vi "Video read with led for 3 part drum.vi"() -> ()   [LabVIEW 2009]
uses:
  <vilib>/vision/Image Controls.llb/IMAQ Image.ctl
  <vilib>/Instr/_visa.llb/VISA Configure Serial Port (Instr).vi
  <vilib>/Analysis/3filter.llb/Filter Passband Type.ctl
  <vilib>/Analysis/3filter.llb/Butterworth Filter (DBL).vi
  <vilib>/vision/NI_Vision_Development_Module.lvlib
  <vilib>/Analysis/NI_AALBase.lvlib
panel:
  in  "ROI Descriptor (Line Profile 2) 3":T1={"Global Rectangle"=[406, 309, 423, 383], "Contours"=[{"ID"=enum."External", "Type"=2, "Coordinates"=[422, 382, 406, 309]}]} {"Contours"."Type" items=["No Selection", "Point", "Line", "Rectangle", "Oval", "Polygon", "Freehand Region", "Annulus", "Unused2", "Unused3", "Broken Line", "Freehand Line", "Rotated Rectangle"]}
  in  "low  3":dbl=0.12500000000000006 format="%0.4f"
  out "Waveform Green":dbl[](graph)
  out "LED Green":bool
  in  "sampling 3":dbl=1.0 format="%0.2f"
  in  "high 3":dbl=60.0 format="%0.2f"
  in  "ROI Descriptor (Line Profile 2)":T1={"Global Rectangle"=[342, 292, 349, 377], "Contours"=[{"ID"=enum."External", "Type"=2, "Coordinates"=[342, 376, 348, 292]}]} {"Contours"."Type" items=["No Selection", "Point", "Line", "Rectangle", "Oval", "Polygon", "Freehand Region", "Annulus", "Unused2", "Unused3", "Broken Line", "Freehand Line", "Rotated Rectangle"]}
  out "Blue Line":T1={"Global Rectangle"=[168, 264, 180, 378], "Contours"=[{"ID"=enum."External", "Type"=2, "Coordinates"=[168, 377, 179, 264]}]} {"Contours"."Type" items=["No Selection", "Point", "Line", "Rectangle", "Oval", "Polygon", "Freehand Region", "Annulus", "Unused2", "Unused3", "Broken Line", "Freehand Line", "Rotated Rectangle"]}
  in  "ROI Descriptor (Line Profile 1) 2":T1={"Global Rectangle"=[376, 303, 382, 378], "Contours"=[{"ID"=enum."External", "Type"=2, "Coordinates"=[376, 303, 381, 377]}]} {"Contours"."Type" items=["No Selection", "Point", "Line", "Rectangle", "Oval", "Polygon", "Freehand Region", "Annulus", "Unused2", "Unused3", "Broken Line", "Freehand Line", "Rotated Rectangle"]}
  out "cluster":T2
  in  "baud rate (9600)":u32=9600
  in  "VISA resource name":refnum<visa-resource-name>
  out "number":u32
  out "decimal integer string":string
  out "Image Dst Out":T3
  out "Yellow Line":T1={"Global Rectangle"=[243, 262, 261, 384], "Contours"=[{"ID"=enum."External", "Type"=2, "Coordinates"=[260, 383, 243, 262]}]} {"Contours"."Type" items=["No Selection", "Point", "Line", "Rectangle", "Oval", "Polygon", "Freehand Region", "Annulus", "Unused2", "Unused3", "Broken Line", "Freehand Line", "Rotated Rectangle"]}
  in  "low  2":dbl=0.12500000000000006 format="%0.4f"
  in  "high 2":dbl=60.0 format="%0.2f"
  in  "sampling 2":dbl=1.0 format="%0.2f"
  out "LED RED":bool
  out "Waveform Yellow":dbl[](graph)
  in  "playtime":dbl=30.0
  out "Frame Number":i32
  in  "Frame Start":i32=2400
  out "LED BLUE":bool
  in  "low":dbl=0.12500000000000006 format="%0.4f"
  out "Waveform Blue":dbl[](graph)
  in  "high":dbl=60.0 format="%0.2f"
  in  "sampling":dbl=1.0 format="%0.2f"
  out "Image":T3(plugin-control)
  in  "stop":bool
  in  "AVI Path":path
  # "RED"
  # "BLUE"
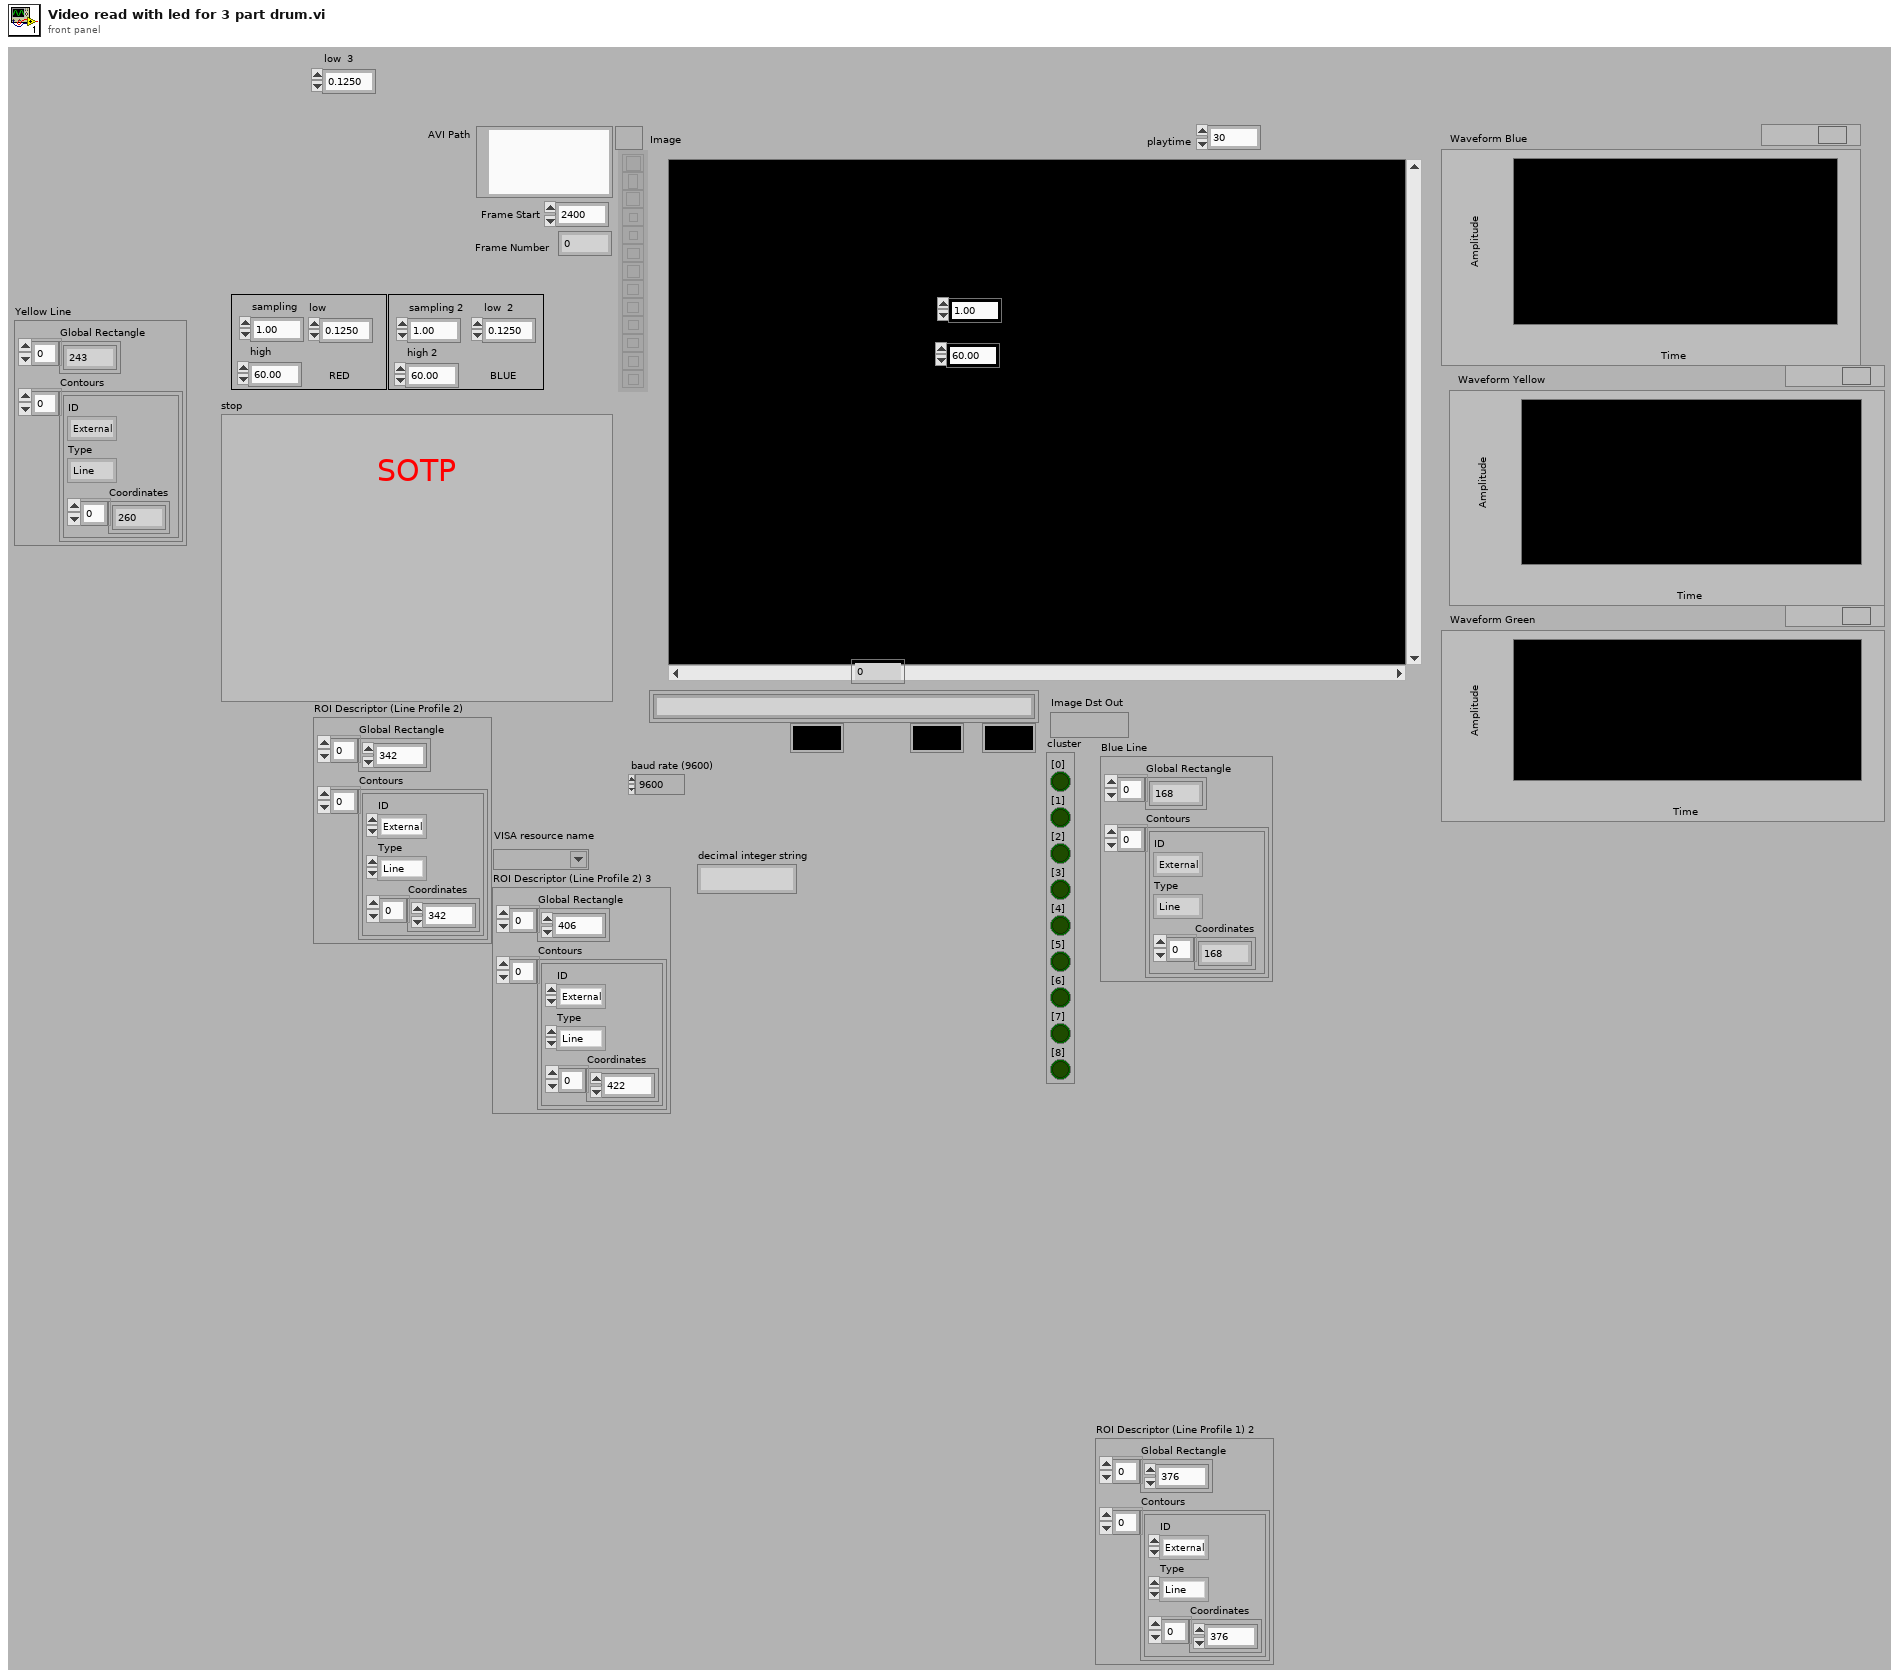
[diagram p1: front panel]
types:
  T1 = cluster{"Global Rectangle":i32[], "Contours":cluster{"ID":enum32{"External", "Internal"}, "Type":u32, "Coordinates":i32[]}[]}
  T2 = cluster{"[0]":bool, "[1]":bool, "[2]":bool, "[3]":bool, "[4]":bool, "[5]":bool, "[6]":bool, "[7]":bool, "[8]":bool}
  T3 = typedef "IMAQ Image.ctl" = refnum<image>
  T4 = typedef "NI_AALBase.lvlib/Filter Passband Type.ctl" = enum32{"Lowpass", "Highpass", "Bandpass", "Bandstop"}
  T5 = cluster{"Left":i32, "Top":i32, "Right":i32, "Bottom":i32}
  T6 = typedef "Image Type" = u32
  T7 = typedef "AviRefnum.ctl" = refnum<k1>
  T8 = cluster{"ID":enum32{"External", "Internal"}, "Type":u32, "Coordinates":i32[]}[]
  T9 = cluster{"ID":enum32{"External", "Internal"}, "Type":u32, "Coordinates":i32[]}
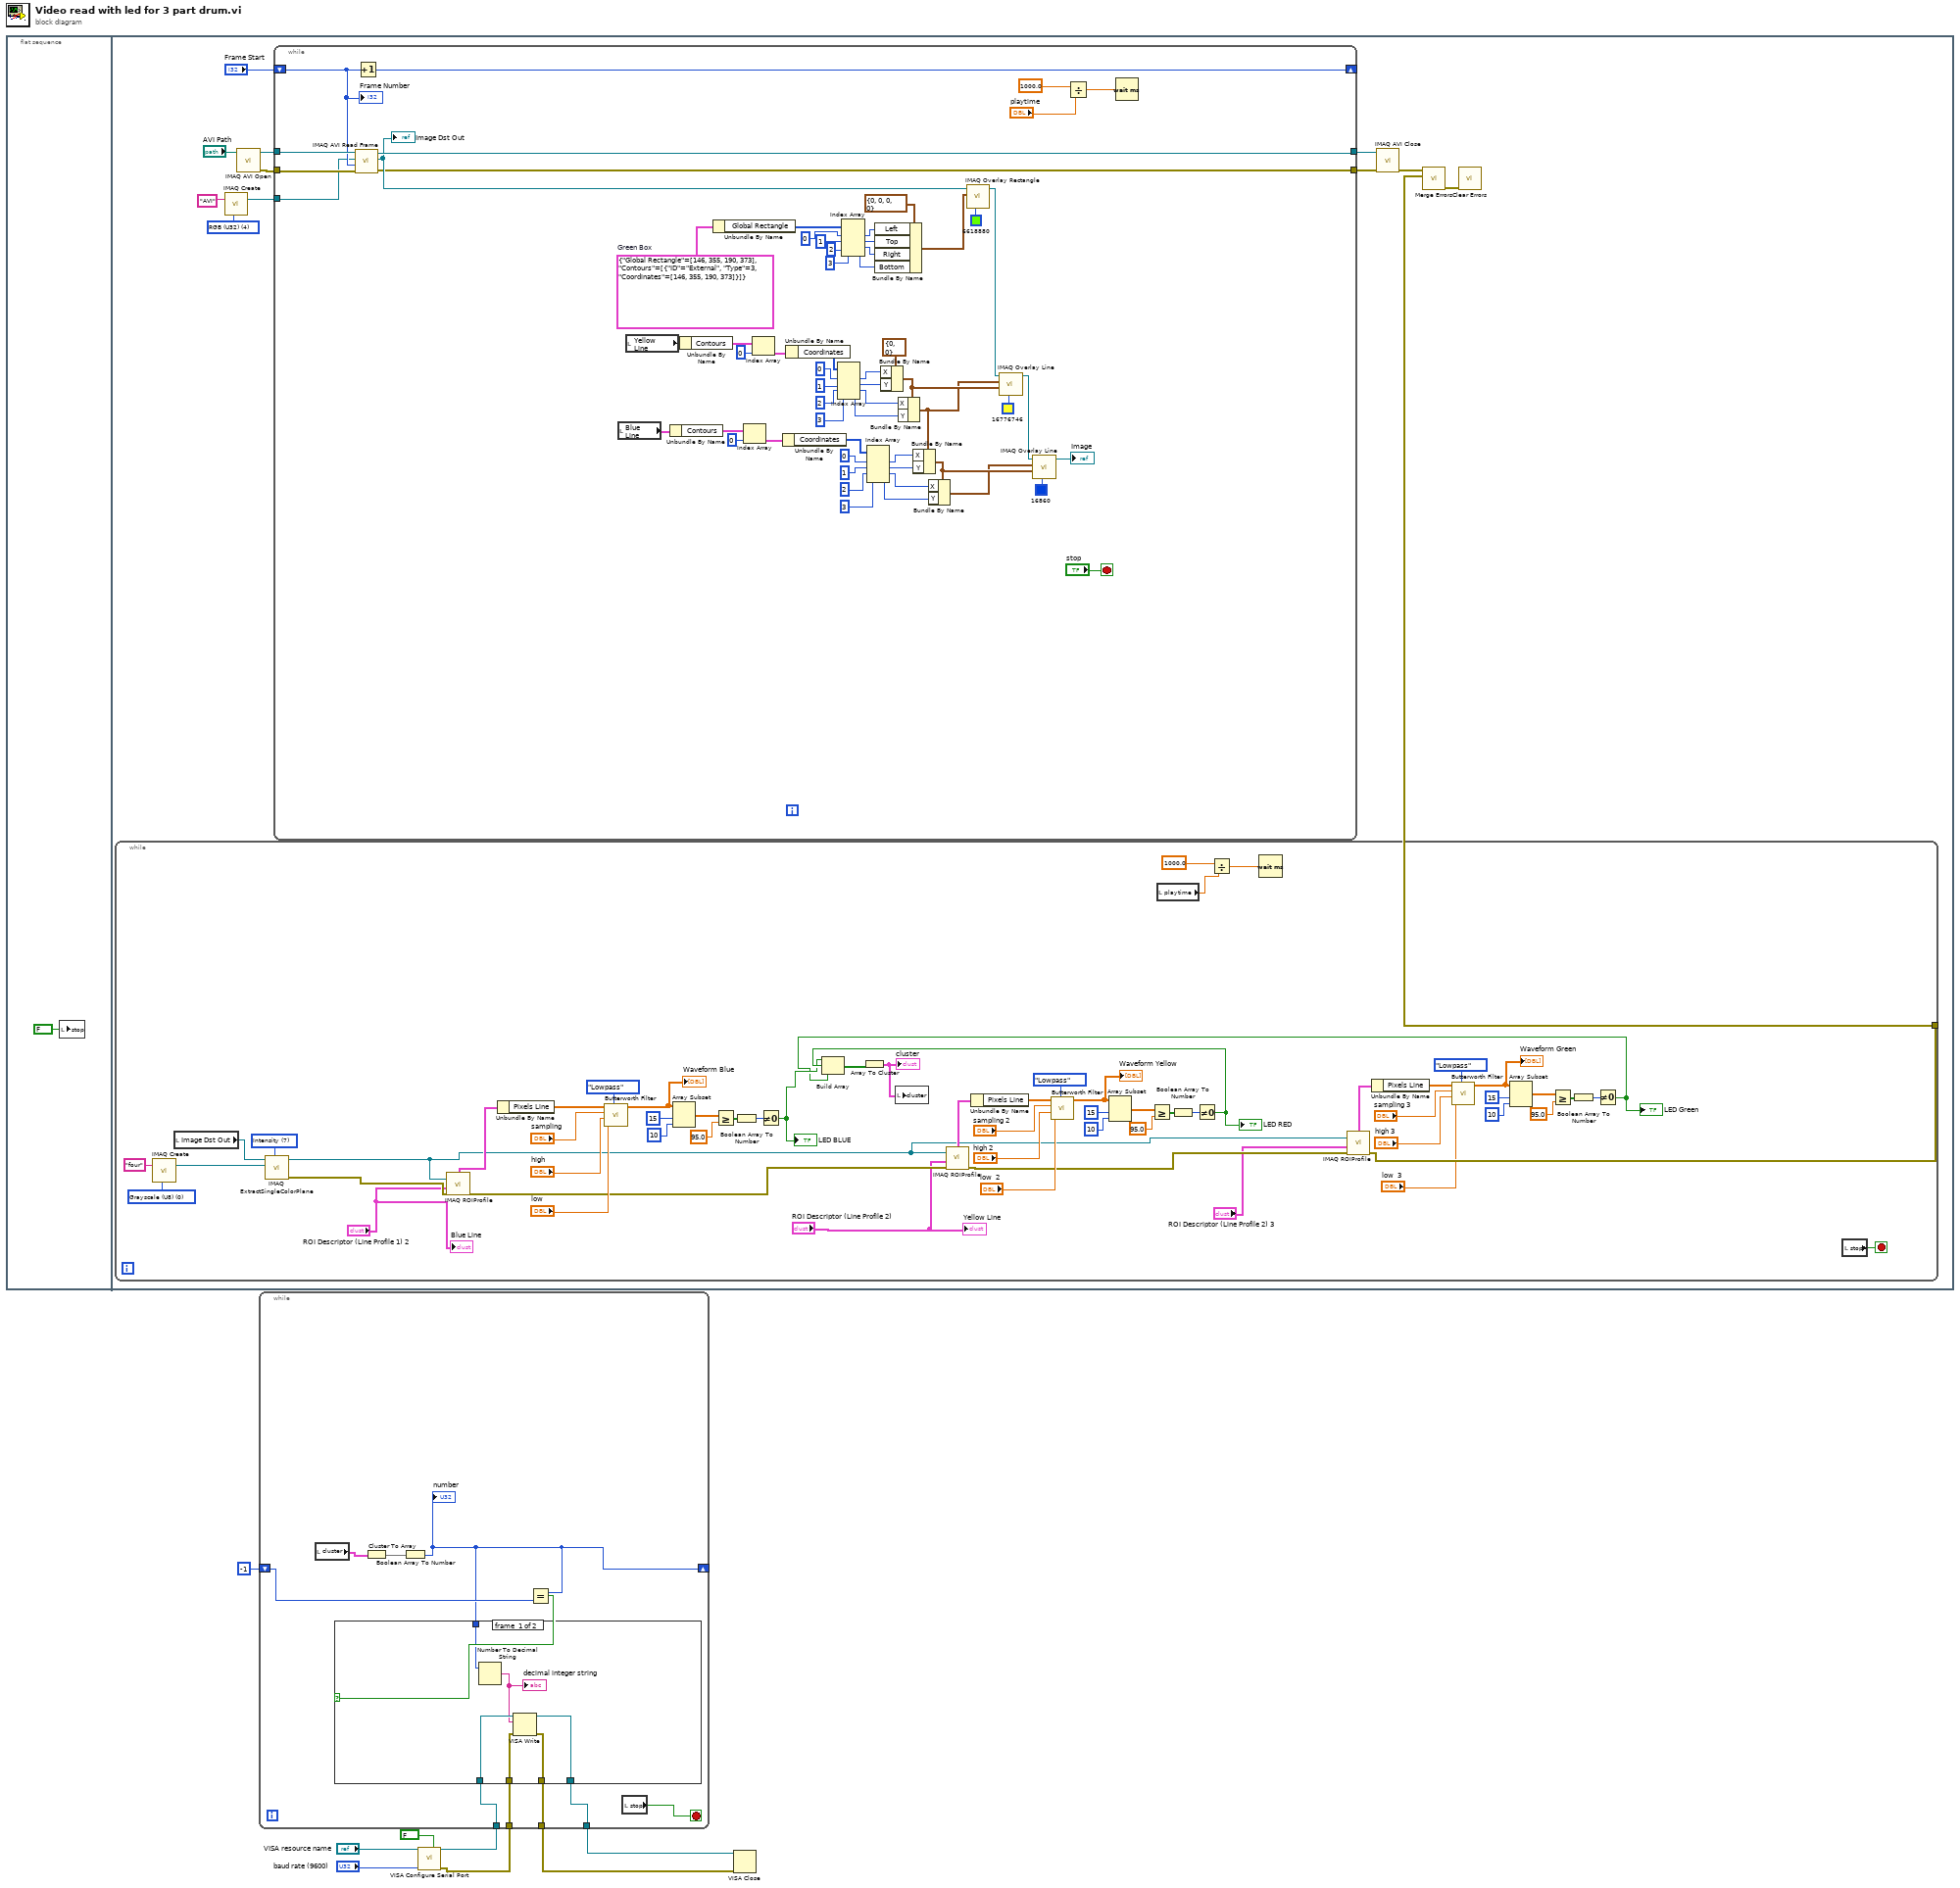
[diagram p0: block diagram]
diagram:
  n1 = flat-sequence {
    frame #0 {
      n2 = local write "stop"(FALSE ("stop")) -> ()
    }
    frame #1 {
      w12 = T6 4 items=["Grayscale (U8)", "Grayscale (I16)", "Grayscale (SGL)", "Complex (CSG)", "RGB (U32)", "HSL (U32)", "RGB (U64)", "Grayscale (U16)"] ("Image Type")
      n3 = while {
        tunnel: [w25] -> w15
        stop <- w81 stop-if-true
        w52 = T6 0 items=["Grayscale (U8)", "Grayscale (I16)", "Grayscale (SGL)", "Complex (CSG)", "RGB (U32)", "HSL (U32)", "RGB (U64)", "Grayscale (U16)"] ("Image Type")
        w82 = 7 items=["Red", "Green", "Blue", "Hue", "Saturation", "Luminance", "Value", "Intensity"] ("Color Plane")
        n4 = call "IMAQ Create"("Image Name"="four", "Image Type"=w52) -> ("New Image"=w50:T3)  [unwired: 3 in, 1 out]
        n5 = local read "Image Dst Out"() -> (w53:T3)
        n6 = call "IMAQ ExtractSingleColorPlane"("Color Plane"=w82, "Image Dst"=w50, "Image Src"=w53) -> ("error out"=w44:errorcluster, "Image Dst Out"=w27:T3)  [unwired: 1 in, 6 out]
        n7 = call "IMAQ ROIProfile"("error in (no error)"=w44, "ROI Descriptor"="ROI Descriptor (Line Profile 1) 2", "Image"=w27) -> ("error out"=w45:errorcluster, "ROI Graph"=w43:cluster{"x0":sgl, "dx":sgl, "Pixels Line":sgl[]})  [unwired: 4 out]
        n8 = Unbundle By Name(w43) -> ("Pixels Line"=w79:sgl[])
        n9 = call-poly <vilib>:"Butterworth Filter.vi"("filter type"=Filter_Passband_Type."Lowpass", "low cutoff freq: fl"="low", "high cutoff freq: fh"="high", "sampling freq: fs"="sampling", "X"=w79) -> ("Filtered X"=w22:dbl[])  [unwired: 3 in, 1 out]
        "Waveform Blue" <- w22
        n10 = Array Subset(array=w22, index=15, length=10) -> (w73:dbl[])
        n11 = Greater Or Equal?(x=w73, y=95.0) -> (x >= y?=w71:bool[])
        n12 = Boolean Array To Number(Boolean array=w71) -> (number=w68:u32)
        n13 = Not Equal To 0?(x=w68) -> (x != 0?=w46:bool)
        "LED BLUE" <- w46
        n14 = call "IMAQ ROIProfile"("error in (no error)"=w45, "ROI Descriptor"="ROI Descriptor (Line Profile 2)", "Image"=w27) -> ("error out"=w26:errorcluster, "ROI Graph"=w56:cluster{"x0":sgl, "dx":sgl, "Pixels Line":sgl[]})  [unwired: 4 out]
        n15 = Unbundle By Name(w56) -> ("Pixels Line"=w59:sgl[])
        n16 = call-poly <vilib>:"Butterworth Filter.vi"("filter type"=Filter_Passband_Type."Lowpass", "low cutoff freq: fl"="low  2", "high cutoff freq: fh"="high 2", "sampling freq: fs"="sampling 2", "X"=w59) -> ("Filtered X"=w55:dbl[])  [unwired: 3 in, 1 out]
        "Waveform Yellow" <- w55
        n17 = Array Subset(array=w55, index=15, length=10) -> (w64:dbl[])
        n18 = Greater Or Equal?(x=w64, y=95.0) -> (x >= y?=w62:bool[])
        n19 = local read "playtime"() -> (w67:dbl)
        n20 = Boolean Array To Number(Boolean array=w62) -> (number=w61:u32)
        n21 = Not Equal To 0?(x=w61) -> (x != 0?=w47:bool)
        "LED RED" <- w47
        n22 = Divide(x=1000.0, y=w67) -> (x/y=w70:dbl)
        n23 = Wait (ms)(milliseconds to wait=w70) -> ()  [unwired: 1 out]
        n24 = call "IMAQ ROIProfile"("error in (no error)"=w26, "ROI Descriptor"="ROI Descriptor (Line Profile 2) 3", "Image"=w27) -> ("error out"=w25:errorcluster, "ROI Graph"=w39:cluster{"x0":sgl, "dx":sgl, "Pixels Line":sgl[]})  [unwired: 4 out]
        n25 = Unbundle By Name(w39) -> ("Pixels Line"=w36:sgl[])
        n26 = call-poly <vilib>:"Butterworth Filter.vi"("filter type"=Filter_Passband_Type."Lowpass", "low cutoff freq: fl"="low  3", "high cutoff freq: fh"="high 3", "sampling freq: fs"="sampling 3", "X"=w36) -> ("Filtered X"=w40:dbl[])  [unwired: 3 in, 1 out]
        "Waveform Green" <- w40
        n27 = Array Subset(array=w40, index=15, length=10) -> (w31:dbl[])
        n28 = Greater Or Equal?(x=w31, y=95.0) -> (x >= y?=w33:bool[])
        n29 = Boolean Array To Number(Boolean array=w33) -> (number=w34:u32)
        n30 = Not Equal To 0?(x=w34) -> (x != 0?=w28:bool)
        "LED Green" <- w28
        n31 = Build Array(w46, w47, w28) -> (w49:bool[])
        n32 = Array To Cluster(array=w49) -> (cluster=w48:T2)
        "cluster" <- w48
        n33 = local write "cluster"(w48) -> ()
        n34 = local read "stop"() -> (w81:bool)
        "Yellow Line" <- "ROI Descriptor (Line Profile 2)"
        "Blue Line" <- "ROI Descriptor (Line Profile 1) 2"
      }
      n35 = call "IMAQ Create"("Image Name"="AVI", "Image Type"=w12) -> ("New Image"=w10:T3)  [unwired: 3 in, 1 out]
      n36 = call "IMAQ AVI Open"("AVI Path"="AVI Path") -> ("error out"=w18:errorcluster, "Avi Refnum"=w19:T7)  [unwired: 9 in]
      n37 = while {
        tunnel: w19 -> [w143]
        tunnel: w18 -> [w88]
        tunnel: [w142] -> w20
        shift-right: [w137] -> _
        shift-left: "Frame Start" -> [w136]
        tunnel: [w84] -> w13
        tunnel: w10 -> [w83]
        stop <- "stop" stop-if-true
        w135 = T1 {"Global Rectangle"=[146, 355, 190, 373], "Contours"=[{"ID"=enum."External", "Type"=3, "Coordinates"=[146, 355, 190, 373]}]}  # Green Box
        n38 = call "IMAQ AVI Read Frame"("error in (no error)"=w88, "Frame Number"=w136, "Image"=w83, "Avi Refnum"=w143) -> ("error out"=w84:errorcluster, "Image Out"=w85:T3, "Avi Refnum (duplicate)"=w142:T7)  [unwired: 4 in, 1 out]
        "Image Dst Out" <- w85
        n39 = Increment(x=w136) -> (x+1=w137:i32)
        n40 = local read "Blue Line"() -> (w87:T1)
        n41 = local read "Yellow Line"() -> (w86:T1)
        n42 = Unbundle By Name(w87) -> ("Contours"=w102:T8)
        n43 = Unbundle By Name(w86) -> ("Contours"=w117:T8)
        n44 = Unbundle By Name(w135) -> ("Global Rectangle"=w131:i32[])
        n45 = Index Array(array=w102, index=0) -> (element=w101:T9)
        n46 = Index Array(array=w117, index=0) -> (element=w119:T9)
        n47 = Unbundle By Name(w101) -> ("Coordinates"=w100:i32[])
        n48 = Unbundle By Name(w119) -> ("Coordinates"=w120:i32[])
        n49 = Index Array(array=w120, index #1=0 ("index"), index #2=1 ("index"), index #3=2 ("index"), index #4=3 ("index")) -> (element #1=w112:i32, element #2=w113:i32, element #3=w114:i32, element #4=w115:i32)
        n50 = Index Array(array=w131, index #1=0 ("index"), index #2=1 ("index"), index #3=2 ("index"), index #4=3 ("index")) -> (element #1=w130:i32, element #2=w129:i32, element #3=w128:i32, element #4=w127:i32)
        n51 = Index Array(array=w100, index #1=0 ("index"), index #2=1 ("index"), index #3=2 ("index"), index #4=3 ("index")) -> (element #1=w99:i32, element #2=w105:i32, element #3=w104:i32, element #4=w103:i32)
        n52 = Bundle By Name(cluster=T5 {"Left"=0, "Top"=0, "Right"=0, "Bottom"=0} ("Rectangle"), "Left"=w130, "Top"=w129, "Right"=w128, "Bottom"=w127) -> (w133:T5)
        n53 = Bundle By Name(cluster=cluster{"X":i32, "Y":i32} {"X"=0, "Y"=0} ("End Point"), "X"=w112, "Y"=w113) -> (w121:cluster{"X":i32, "Y":i32})
        n54 = Bundle By Name(cluster=w121, "X"=w114, "Y"=w115) -> (w91:cluster{"X":i32, "Y":i32})
        n55 = Bundle By Name(cluster=w91, "X"=w99, "Y"=w105) -> (w106:cluster{"X":i32, "Y":i32})
        n56 = Bundle By Name(cluster=w106, "X"=w104, "Y"=w103) -> (w97:cluster{"X":i32, "Y":i32})
        n57 = call "IMAQ Overlay Rectangle"("Color"=u32 6618880, "Rectangle"=w133, "Image"=w85) -> ("Image Out"=w107:T3)  [unwired: 7 in, 1 out]
        n58 = call "IMAQ Overlay Line"("Color"=u32 16776746, "End Point"=w121, "Start Point"=w91, "Image"=w107) -> ("Image Out"=w96:T3)  [unwired: 6 in, 1 out]
        n59 = call "IMAQ Overlay Line"("Color"=u32 16860, "End Point"=w106, "Start Point"=w97, "Image"=w96) -> ("Image Out"=→"Image":T3)  [unwired: 6 in, 1 out]
        n60 = Divide(x=1000.0, y="playtime") -> (x/y=w140:dbl)
        n61 = Wait (ms)(milliseconds to wait=w140) -> ()  [unwired: 1 out]
        "Frame Number" <- w136
      }
      n62 = call "IMAQ AVI Close"("error in (no error)"=w13, "Avi Refnum"=w20) -> ("error out"=w16:errorcluster)  [unwired: 9 in]
      n63 = call <vilib>:"Merge Errors.vi"("error in 2 (no error)"=w15, "error in 1 (no error)"=w16) -> ("error out"=w14:errorcluster)  [unwired: 5 in]
      n64 = call <vilib>:"Clear Errors.vi"("error in (no error)"=w14) -> ()  [unwired: 6 in, 1 out]
    }
  }
  n65 = call-poly "VISA Configure Serial Port"("VISA resource name"="VISA resource name", "Enable Termination\nChar (T)"=FALSE ("Enable Termination\nChar (T)"), "baud rate (9600)"="baud rate (9600)") -> ("VISA resource name out"=w7:refnum<visa-resource-name>, "error out"=w2:errorcluster)  [unwired: 11 in]
  n66 = while {
    shift-right: [w147] -> _
    shift-left: -1 -> [w153]
    tunnel: w7 -> [w151]
    tunnel: [w150] -> w6
    tunnel: w2 -> [w149]
    tunnel: [w148] -> w1
    stop <- w144 stop-if-true
    n67 = local read "cluster"() -> (w145:T2)
    n68 = Cluster To Array(cluster=w145) -> (array=w146:bool[])
    n69 = Boolean Array To Number(Boolean array=w146) -> (number=w147:u32)
    "number" <- w147
    n70 = Equal?(x=w147, y=w153) -> (x = y?=w152:bool)
    n71 = case shown="False" w152 {
      tunnel: w151 -> [w159 w161]
      tunnel: [w158 w161] -> w150
      tunnel: w147 -> [w156 _]
      tunnel: w149 -> [w155 w160]
      tunnel: [w154 w160] -> w148
      frame #0 {
        n72 = Number To Decimal String(number=w156) -> (decimal integer string=w157:string)  [unwired: 1 in]
        "decimal integer string" <- w157
        n73 = VISA Write(VISA resource name=w159, write buffer=w157, error in (no error)=w155) -> (VISA resource name out=w158:refnum<visa-resource-name>, error out=w154:errorcluster)  [unwired: 1 out]
      }
      frame #1 {
      }
    }
    n74 = local read "stop"() -> (w144:bool)
  }
  n75 = VISA Close(VISA resource name=w6, error in (no error)=w1) -> ()  [unwired: 1 out]
